vi "VCI Set Reference.vi"(6 "pData":u32, 7 "RefType":u32, 8 "error in (no error)":errorcluster, 9 "CANIndex":u32, 10 "DevIndex":u32, 11 "DevType":u32) -> (0 "error out":errorcluster, 3 "function return":u32, 4 "pData out":u32)   [LabVIEW 2012, in "ControlCAN.lvlib"]
doc: "unsigned int WINAPI VCI_SetReference(unsigned int DevType,unsigned int DevIndex,unsigned int CANIndex,unsigned int RefType,void *pData);"
uses:
  ControlCAN.lvlib
  Ginkgo_Driver.dll
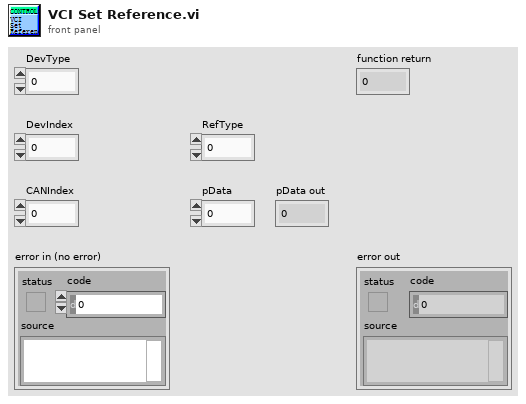
[diagram p1: front panel]
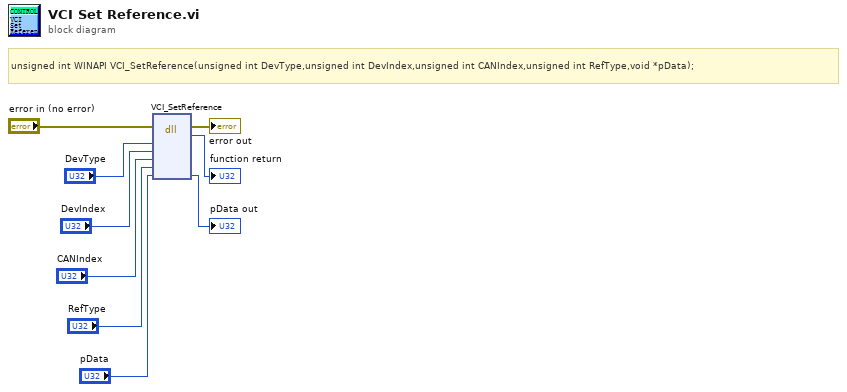
[diagram p0: block diagram]
diagram:
  # "unsigned int WINAPI VCI_SetReference(unsigned int DevType,unsigned int DevIndex,unsigned int CANIndex,unsigned int RefType,void *pData);"
  n1 = dll-call lib="E:/Project/vt_ginkgo/truck/Ginkgo Driver/vs2010/Ginkgo_USB-I2C_API_v2.0.3.0/lib/labview_32bit/ControlCAN/Ginkgo_Driver.*" fn="VCI_SetReference"(error in="error in (no error)", "DevType"="DevType", "DevIndex"="DevIndex", "CANIndex"="CANIndex", "RefType"="RefType", "pData"="pData") -> (error out=→"error out":errorcluster, →"function return":u32, "pData"=→"pData out":u32)  [unwired: 6 in, 1 out]
